vi "Event_kick.vi"(8 "error in (no error)":errorcluster, 10 "Game":refnum<class "Game.lvclass">, 11 "Events in":refnum<class "Events.lvclass">) -> (0 "error out":errorcluster, 2 "kick":bool, 3 "Events out":refnum<class "Events.lvclass">)   [LabVIEW 2023, in "Events.lvclass"]
uses:
  Events.lvclass
  Game_class/Game.lvclass
  Events.lvclass/Events.ctl
  Game_class/Game.lvclass/Game.ctl
  Object_class/Object.lvclass/Object.ctl
  Game_class/Read BallRef.vi
  Game_class/Read Utilities.lvclass.vi
  Object_class/Read x.vi
  Object_class/Read y.vi
  Read touch.vi
  Write kick.vi
  Ball_class/Ball.lvclass
  Utilities_class/Utilities.lvclass
panel:
  out "Boolean":bool
  in  "Dist":dbl=100.0
  in  "Time":u32=100
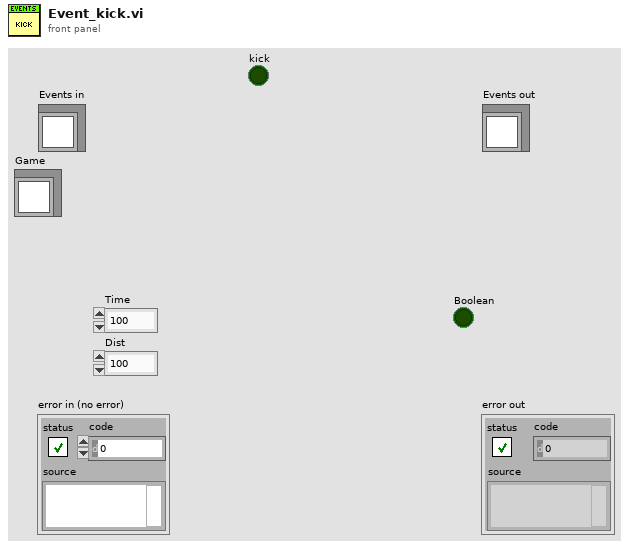
[diagram p1: front panel]
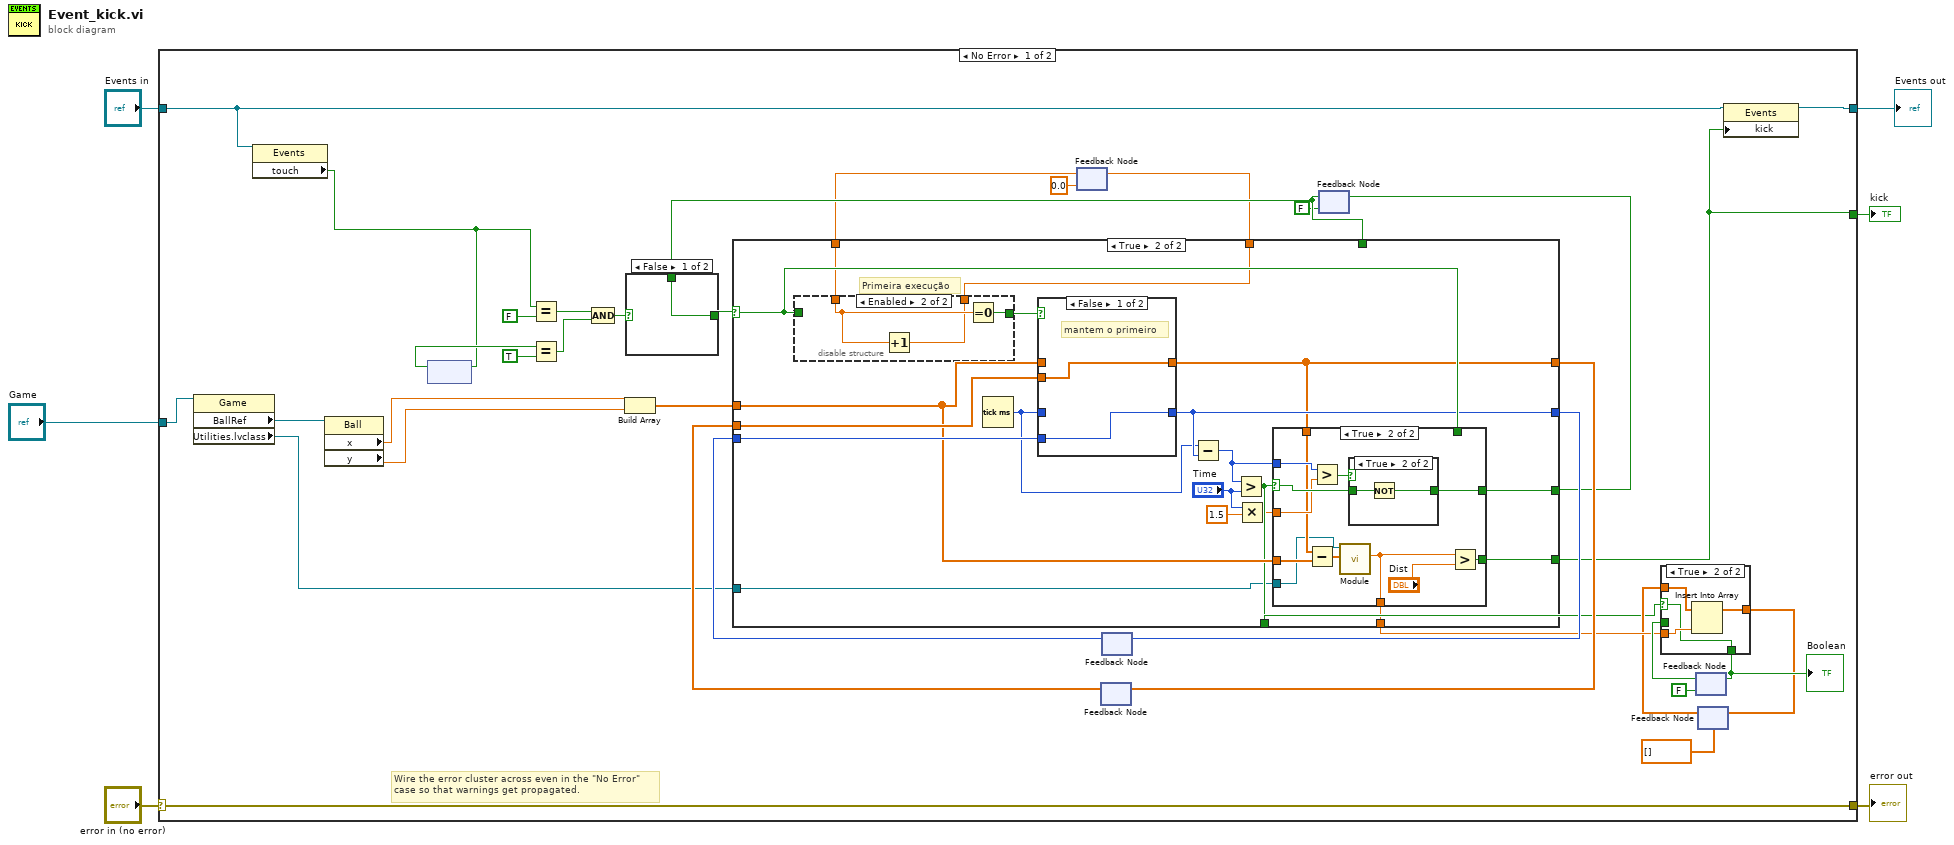
[diagram p0: block diagram]
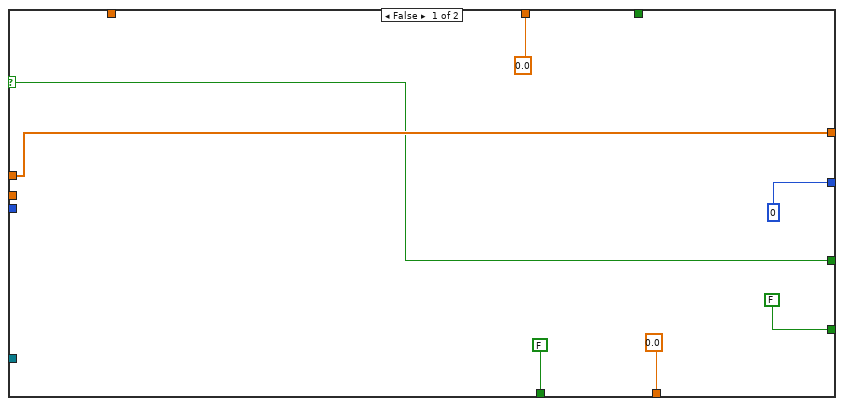
[diagram p4: hidden frame]
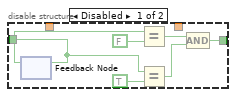
[diagram p5: hidden frame]
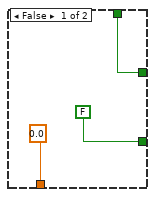
[diagram p6: hidden frame]
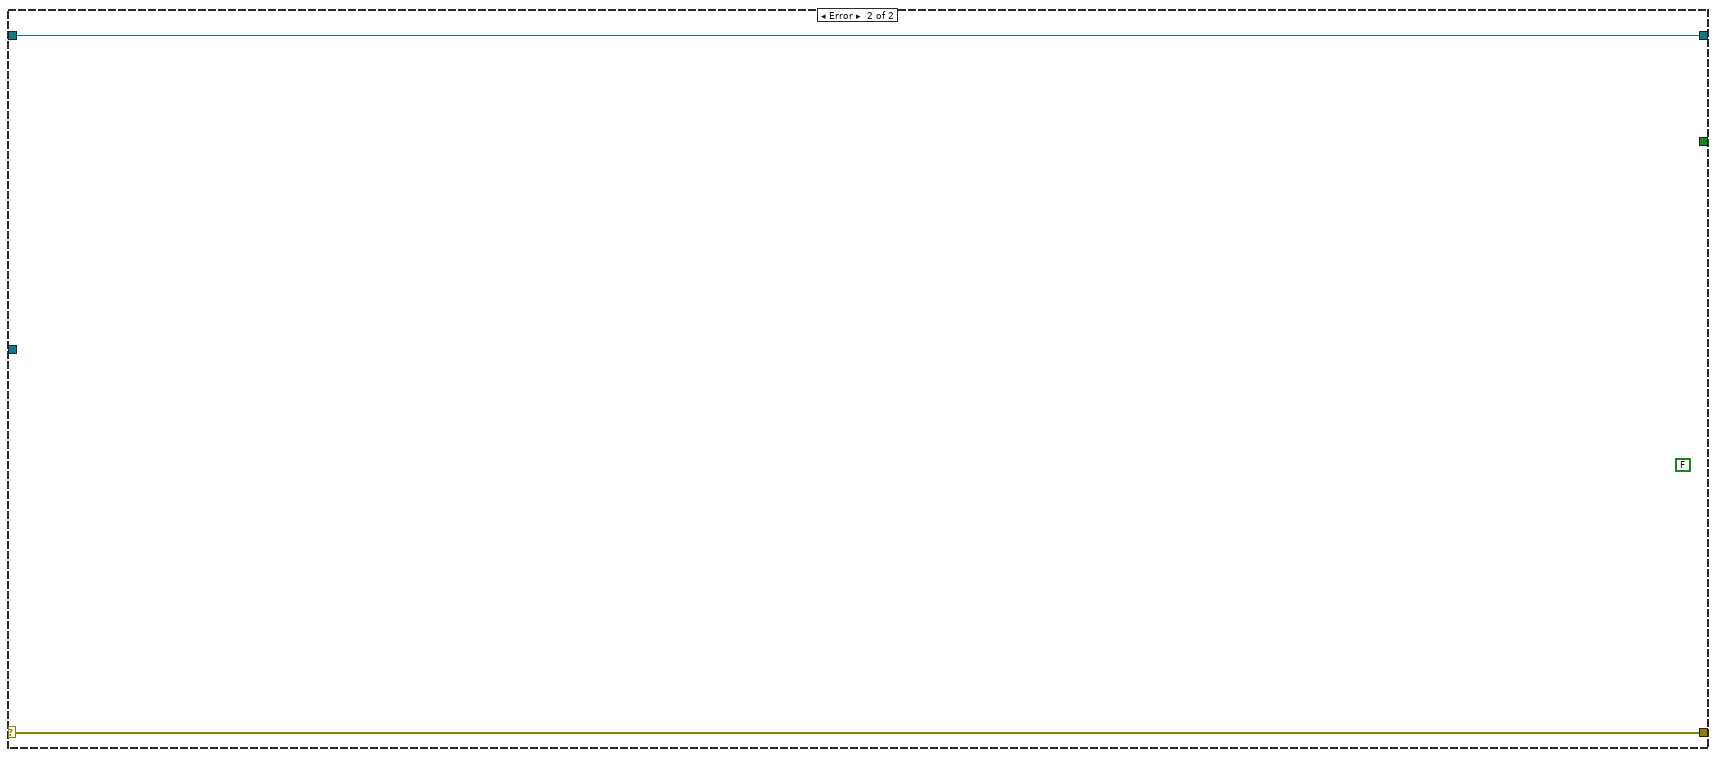
[diagram p9: hidden frame]
diagram:
  n1 = case shown="No Error" "error in (no error)" {
    selector: "error in (no error)" -> [w42 w110]
    tunnel: [w42 w110] -> w5
    tunnel: [w11 w109] -> w3
    tunnel: "Events in" -> [w9 w109]
    tunnel: "Game" -> [w15 _]
    tunnel: [w7 _] -> w1
    frame No Error {
      # "Wire the error cluster across even in the \"No Error\"\ncase so that warnings get propagated."
      n2 = property class="Game"(reference=w15) -> ("BallRef"=w14:refnum<class "Ball.lvclass">, "Utilities.lvclass"=w10:refnum<class "Utilities.lvclass">)  [unwired: 1 in, 2 out]
      n3 = property class="Events"(reference=w9) -> ("touch"=w8:bool)  [unwired: 1 in, 2 out]
      n4 = property class="Ball"(reference=w14) -> ("x"=w13:dbl, "y"=w12:dbl)  [unwired: 1 in, 2 out]
      n5 = feedback #1() -> (w39:bool)  [unwired: 1 in]
      n6 = feedback-in #1(w8) -> ()
      n7 = Equal?(x=w8, y=FALSE) -> (x = y?=w41:bool)
      n8 = Equal?(x=w39, y=TRUE) -> (x = y?=w40:bool)
      n9 = Compound Arithmetic op=AND(w41, w40) -> (w29:bool)
      n10 = Build Array(w13, w12) -> (w36:dbl[])
      n11 = feedback #2(0.0 ("Numeric")) -> (w18:dbl)
      n12 = feedback #3() -> (w34:dbl[])  [unwired: 1 in]
      n13 = feedback #4() -> (w32:u32)  [unwired: 1 in]
      n14 = feedback #5(FALSE) -> (w30:bool)
      n15 = case shown="False" w29 {
        selector: w29 -> [_ w50]
        tunnel: w30 -> [w49 _]
        tunnel: [w49 w50] -> w28
        frame False {
        }
        frame True {
        }
      }
      n16 = case shown="True" w28 {
        selector: w28 -> [w54 w76]
        tunnel: w36 -> [w57 w72]
        tunnel: [w57 w71] -> w35
        tunnel: w34 -> [_ w75]
        tunnel: [u32 0 ("millisecond timer value") w73] -> w33
        tunnel: w32 -> [_ w74]
        tunnel: [FALSE w70] -> w7
        tunnel: [w54 w69] -> w31
        tunnel: w30 -> [_ _]
        tunnel: [0.0 ("Modulo") w68] -> w23
        tunnel: [FALSE w67] -> w19
        tunnel: w18 -> [_ w66]
        tunnel: [0.0 w65] -> w16
        tunnel: w10 -> [_ w58]
        frame False {
        }
        frame True {
          # "Primeira execução"
          n17 = disable-structure shown="Enabled" {
            disable-tunnel: [w78 w86] -> w64
            disable-tunnel: w76 -> [w77 _]
            disable-tunnel: w66 -> [_ w85]
            disable-tunnel: [_ w84] -> w65
            frame Disabled {
              n18 = feedback #6() -> (w79:bool)  [unwired: 1 in]
              n19 = feedback-in #6(w77) -> ()
              n20 = Equal?(x=w79, y=FALSE) -> (x = y?=w83:bool)
              n21 = Equal?(x=w77, y=TRUE) -> (x = y?=w82:bool)
              n22 = Compound Arithmetic op=AND(w83, w82) -> (w78:bool)
            }
            frame Enabled {
              n23 = Increment(x=w85) -> (x+1=w84:dbl)
              n24 = Equal To 0?(x=w85) -> (x = 0?=w86:bool)
            }
          }
          n25 = Tick Count (ms)() -> (millisecond timer value=w63:u32)
          n26 = case shown="False" w64 {
            tunnel: w72 -> [_ w108]
            tunnel: [w106 w108] -> w71
            tunnel: w75 -> [w106 _]
            tunnel: [w105 w107] -> w73
            tunnel: w63 -> [_ w107]
            tunnel: w74 -> [w105 _]
            frame False {
              # "mantem o primeiro"
            }
            frame True {
              # "atualiza o valor do \nprimeiro"
            }
          }
          n27 = Subtract(x=w63, y=w73) -> (x-y=w62:u32)
          n28 = Greater?(x=w62, y="Time") -> (0:w67:bool)
          n29 = Multiply(x="Time", y=1.5) -> (x*y=w59:dbl)
          n30 = case shown="True" w67 {
            selector: w67 -> [_ w99]
            tunnel: w72 -> [_ w93]
            tunnel: w71 -> [_ w94]
            tunnel: [FALSE w100] -> w70
            tunnel: [w88 w98] -> w69
            tunnel: w76 -> [w88 _]
            tunnel: [0.0 ("Modulo") w91] -> w68
            tunnel: w62 -> [_ w97]
            tunnel: w59 -> [_ w96]
            tunnel: w58 -> [_ w90]
            frame False {
            }
            frame True {
              n31 = Subtract(x=w94, y=w93) -> (x-y=w92:dbl[])
              n32 = Greater?(x=w97, y=w96) -> (0:w95:bool)
              n33 = call "Module.vi"("2D vector"=w92, "Utilities in"=w90) -> ("Modulo"=w91:dbl)  [unwired: 7 in, 2 out]
              n34 = case shown="True" w95 {
                tunnel: w99 -> [w102 w104]
                tunnel: [w102 w103] -> w98
                frame False {
                }
                frame True {
                  n35 = Not(x=w104) -> (.not. x?=w103:bool)
                }
              }
              n36 = Greater?(x=w91, y="Dist") -> (0:w100:bool)
            }
          }
        }
      }
      n37 = feedback-in #2(w16) -> ()
      n38 = feedback-in #3(w35) -> ()
      n39 = feedback-in #4(w33) -> ()
      n40 = feedback-in #5(w31) -> ()
      n41 = feedback #7(FALSE) -> (w25:bool)
      n42 = feedback #8(dbl[] []) -> (w21:dbl[])
      n43 = case shown="True" w19 {
        selector: w19 -> [_ w45]
        tunnel: [w43 w45] -> w26
        tunnel: w25 -> [w43 _]
        tunnel: w23 -> [_ w48]
        tunnel: [w44 w47] -> w22
        tunnel: w21 -> [w44 w46]
        frame False {
        }
        frame True {
          n44 = Insert Into Array(array=w46, new element=w48) -> (w47:dbl[])  [unwired: 1 in]
        }
      }
      "Boolean" <- w26
      n45 = feedback-in #7(w26) -> ()
      n46 = feedback-in #8(w22) -> ()
      n47 = property class="Events"(reference=w9, "kick"=w7) -> (reference out=w11:refnum<class "Events.lvclass">)  [unwired: 1 in, 1 out]
    }
    frame Error {
      (unwired) FALSE
    }
  }
  "error out" <- w5
  "Events out" <- w3
  "kick" <- w1
